vi "Error URI.vi"(11 "ErrorOrSuccess JSON in":refnum<class "ErrorOrSuccess JSON.lvclass">) -> (2 "Error URI":string, 3 "ErrorOrSuccess JSON out":refnum<class "ErrorOrSuccess JSON.lvclass">)   [LabVIEW 2020, in "wamplv.lvlib" / "ErrorOrSuccess JSON.lvclass"]
uses:
  ErrorOrSuccess JSON.lvclass
  ErrorOrSuccess JSON.lvclass/ErrorOrSuccess JSON.ctl
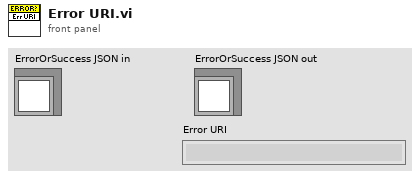
[diagram p1: front panel]
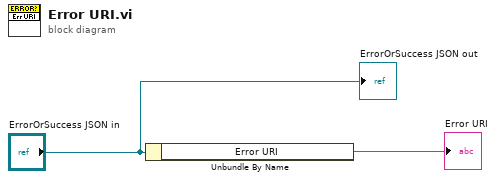
[diagram p0: block diagram]
diagram:
  n1 = Unbundle By Name("ErrorOrSuccess JSON in") -> ("Error URI"=→"Error URI":string)
  "ErrorOrSuccess JSON out" <- "ErrorOrSuccess JSON in"
